vi "piezoWriteCloseNew.vi"   [LabVIEW 2017]
uses:
  globalDevices.vi
  <vilib>/DAQmx/create/channels.llb/DAQmx Create Channel (AO-Voltage-Basic).vi
  <vilib>/DAQmx/create/channels.llb/DAQmx Create Channel (AI-Voltage-Basic).vi
  <vilib>/DAQmx/read.llb/DAQmx Read (Analog DBL 1Chan 1Samp).vi
  <vilib>/DAQmx/write.llb/DAQmx Write (Analog DBL 1Chan 1Samp).vi
  Piezo/lvlib/Madlib.lvlib
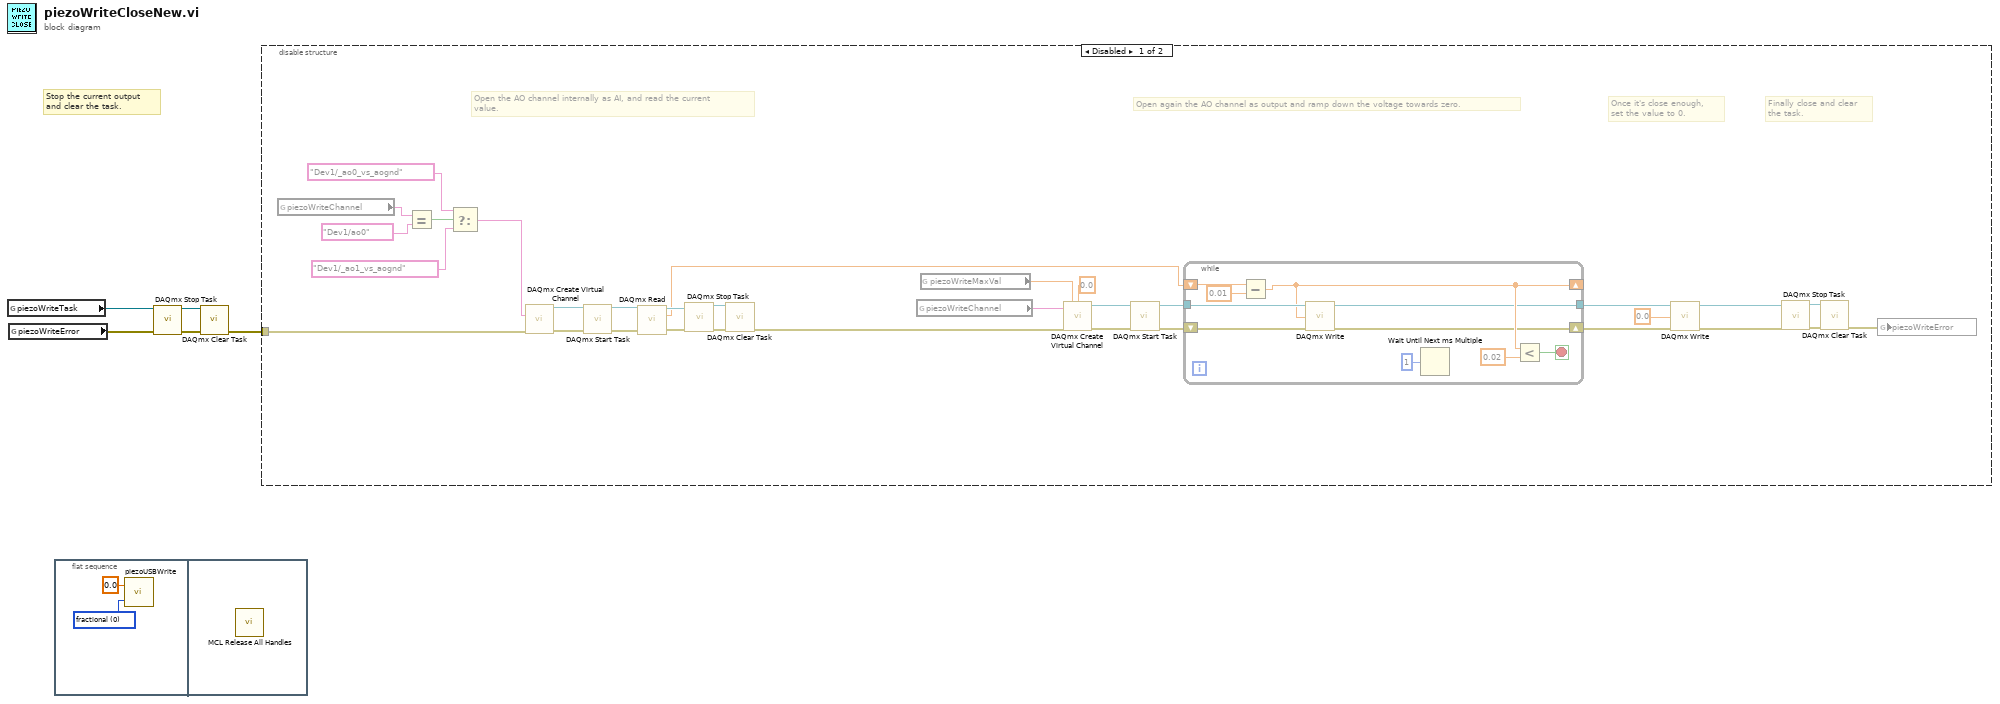
[diagram p0: block diagram]
diagram:
  # "Stop the current output\nand clear the task."
  n1 = global read "globalDevices.vi" "piezoWriteTask"() -> (w4:refnum<k21>)
  n2 = global read "globalDevices.vi" "piezoWriteError"() -> (w5:errorcluster)
  n3 = flat-sequence {
    frame #0 {
      w6 = u16 0 items=["fractional", "voltage (V)", "position (um)"] ("mode")
      n4 = call "piezoUSBWrite.vi"("mode"=w6, "position"=0.0) -> ()  [unwired: 1 in]
    }
    frame #1 {
      n5 = call "MCL Release All Handles.vi"() -> ()  [unwired: 12 in]
    }
  }
  n6 = call <vilib>:"DAQmx Stop Task.vi"("task/channels in"=w4, "error in"=w5) -> ("task out"=w2:refnum<k21>, "error out"=w3:errorcluster)  [unwired: 12 in]
  n7 = call <vilib>:"DAQmx Clear Task.vi"("task in"=w2, "error in"=w3) -> ("error out"=w1:errorcluster)  [unwired: 13 in]
  n8 = disable-structure shown="Disabled" {
    disable-tunnel: w1 -> [w19 _]
    frame Disabled {
      # "Finally close and clear\nthe task."
      # "Once it's close enough,\nset the value to 0."
      # "Open again the AO channel as output and ramp down the voltage towards zero."
      # "Open the AO channel internally as AI, and read the current\nvalue."
      n9 = global read "globalDevices.vi" "piezoWriteChannel"() -> (w25:tag)
      n10 = Equal?(x=w25, y=tag "Dev1/ao0" ("physical channels")) -> (x = y?=w23:bool)
      n11 = Select(t=tag "Dev1/_ao0_vs_aognd" ("physical channels"), s=w23, f=tag "Dev1/_ao1_vs_aognd" ("physical channels")) -> (s? t:f=w20:tag)
      n12 = call-poly <vilib>:"DAQmx Create Virtual Channel.vi"("physical channels"=w20, "error in"=w19) -> ("task out"=w31:refnum<k21>, "error out"=w18:errorcluster)  [unwired: 12 in]
      n13 = call <vilib>:"DAQmx Start Task.vi"("task/channels in"=w31, "error in"=w18) -> ("task out"=w30:refnum<k21>, "error out"=w17:errorcluster)  [unwired: 12 in]
      n14 = call-poly <vilib>:"DAQmx Read.vi"("task/channels in"=w30, "error in"=w17) -> ("task out"=w29:refnum<k21>, "data"=w27:dbl, "error out"=w16:errorcluster)  [unwired: 11 in]
      n15 = call <vilib>:"DAQmx Stop Task.vi"("task/channels in"=w29, "error in"=w16) -> ("task out"=w33:refnum<k21>, "error out"=w32:errorcluster)  [unwired: 12 in]
      n16 = call <vilib>:"DAQmx Clear Task.vi"("task in"=w33, "error in"=w32) -> ("error out"=w28:errorcluster)  [unwired: 13 in]
      n17 = global read "globalDevices.vi" "piezoWriteChannel"() -> (w26:tag)
      n18 = global read "globalDevices.vi" "piezoWriteMaxVal"() -> (w34:dbl)
      n19 = call-poly <vilib>:"DAQmx Create Virtual Channel.vi"("maximum value"=w34, "minimum value"=0.0, "physical channels"=w26, "error in"=w28) -> ("task out"=w36:refnum<k21>, "error out"=w15:errorcluster)  [unwired: 10 in]
      n20 = call <vilib>:"DAQmx Start Task.vi"("task/channels in"=w36, "error in"=w15) -> ("task out"=w35:refnum<k21>, "error out"=w14:errorcluster)  [unwired: 12 in]
      n21 = while {
        shift-right: [w44] -> _
        shift-left: w27 -> [w49]
        tunnel: w35 -> [w45]
        tunnel: [w43] -> w13
        shift-right: [w40] -> w12
        shift-left: w14 -> [w41]
        stop <- w46 stop-if-true
        n22 = Subtract(x=w49, y=0.01) -> (x-y=w44:dbl)
        n23 = call-poly <vilib>:"DAQmx Write.vi"("task/channels in"=w45, "data"=w44, "error in"=w41) -> ("task out"=w43:refnum<k21>, "error out"=w40:errorcluster)  [unwired: 10 in, 1 out]
        n24 = Wait Until Next ms Multiple(millisecond multiple=u32 1) -> ()  [unwired: 1 out]
        n25 = Less?(x=w44, y=0.02) -> (x < y?=w46:bool)
      }
      n26 = call-poly <vilib>:"DAQmx Write.vi"("task/channels in"=w13, "data"=0.0, "error in"=w12) -> ("task out"=w11:refnum<k21>, "error out"=w10:errorcluster)  [unwired: 10 in, 1 out]
      n27 = call <vilib>:"DAQmx Stop Task.vi"("task/channels in"=w11, "error in"=w10) -> ("task out"=w39:refnum<k21>, "error out"=w38:errorcluster)  [unwired: 12 in]
      n28 = call <vilib>:"DAQmx Clear Task.vi"("task in"=w39, "error in"=w38) -> ("error out"=w8:errorcluster)  [unwired: 13 in]
      n29 = global write "globalDevices.vi" "piezoWriteError"(w8) -> ()
    }
    frame Enabled {
    }
  }
